vi "jsonDeleteKey.vi"(8 "error in (no error)":errorcluster, 10 "path":string, 11 "d in":i64) -> (0 "error out":errorcluster, 1 "found?":bool, 3 "d out":i64)   [LabVIEW 2016, in "JSON Document.lvclass"]
uses:
  API/JSON Document Class/JSON Document.lvclass
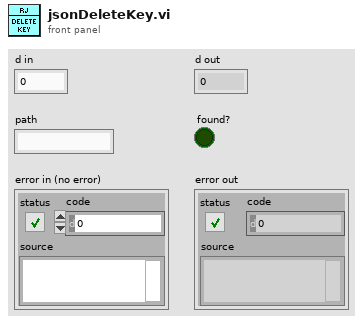
[diagram p1: front panel]
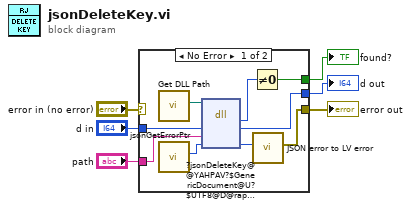
[diagram p0: block diagram]
diagram:
  n1 = case shown="No Error" "error in (no error)" {
    selector: "error in (no error)" -> [_ w17]
    tunnel: [w12 w17] -> w6
    tunnel: "d in" -> [w11 w16]
    tunnel: [w10 w16] -> w3
    tunnel: "path" -> [w9 _]
    tunnel: [w7 _] -> w1
    frame No Error {
      n2 = call "Get DLL Path.vi"() -> ("Path"=w15:path)  [unwired: 11 in]
      n3 = call "jsonGetErrorPtr.vi"() -> ("return type"=w14:i64)  [unwired: 10 in, 1 out]
      n4 = dll-call lib="C:/Users/tblair/Documents/Git Projects/LVrapidjson core/lvrjs/Debug/lvrjs.dll" fn="?jsonDeleteKey@@YAHPAV?$GenericDocument@U?$UTF8@D@rapidjson@@V?$MemoryPoolAllocator@VCrtAllocator@rapidjson@@@2@VCrtAllocator@2@@rapidjson@@PAD0@Z"(path in=w15, "d"=w11, "path"=w9, "jsonError"=w14) -> ("return type"=w8:i32, "d"=w10:i64, "jsonError"=w13:i64)  [unwired: 3 in, 2 out]
      n5 = Not Equal To 0?(x=w8) -> (x != 0?=w7:bool)
      n6 = call "JSON error to LV error.vi"("jsonError"=w13) -> ("error out"=w12:errorcluster)  [unwired: 10 in]
    }
    frame Error {
    }
  }
  "error out" <- w6
  "d out" <- w3
  "found?" <- w1
